vi "Get Name Filtered Categories.vi"(8 "error in (no error)":errorcluster, 10 "Name filter":string, 11 "Database in":refnum<class "Account History.lvclass">) -> (0 "error out":errorcluster, 2 "Categories":refnum<class "Category.lvclass">[](array[class]), 3 "Database out":refnum<class "Account History.lvclass">)   [LabVIEW 2018, in "Account History.lvclass"]
uses:
  Account History.lvclass
  Category/Category.lvclass
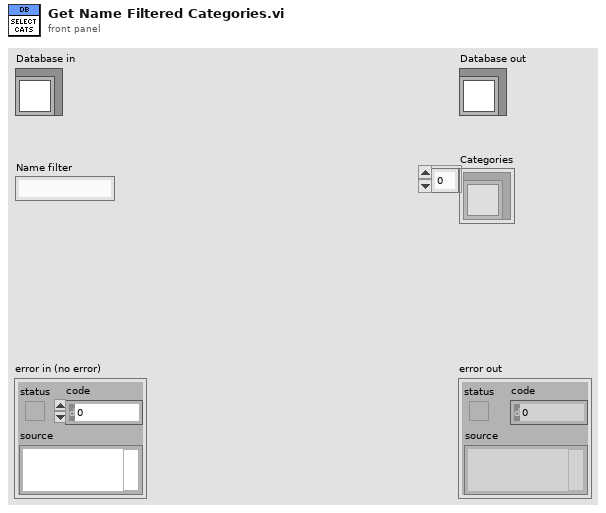
[diagram p1: front panel]
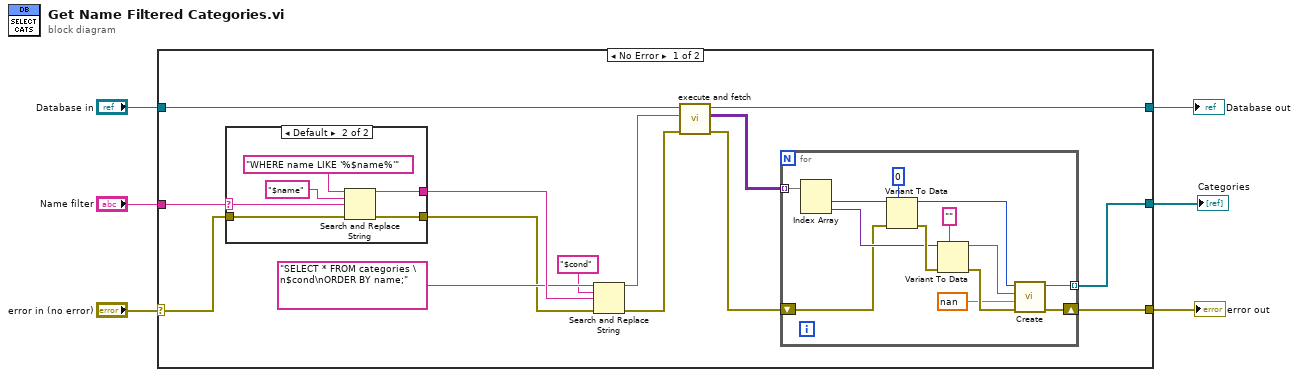
[diagram p0: block diagram]
diagram:
  n1 = case shown="No Error" "error in (no error)" {
    selector: "error in (no error)" -> [w8 w41]
    tunnel: [w13 w42] -> w6
    tunnel: "Database in" -> [w12 w42]
    tunnel: [w11 w41] -> w4
    tunnel: "Name filter" -> [w10 _]
    tunnel: [w9 _] -> w2
    frame No Error {
      n2 = case shown="Default" w10 {
        selector: w10 -> [_ w27]
        tunnel: [_ w24] -> w17
        tunnel: w8 -> [w21 w23]
        tunnel: [w21 w22] -> w7
        frame "" {
        }
        frame Default {
          n3 = Search and Replace String(input string="WHERE name LIKE '%$name%'", search string="$name", replace string=w27, error in=w23) -> (result string=w24:string, error out=w22:errorcluster)  [unwired: 4 in, 2 out]
        }
      }
      n4 = Search and Replace String(input string="SELECT * FROM categories \n$cond\nORDER BY name;", search string="$cond", replace string=w17, error in=w7) -> (result string=w14:string, error out=w18:errorcluster)  [unwired: 4 in, 2 out]
      n5 = call "execute and fetch.vi"("error in (no error)"=w18, "SQL query"=w14, "Database in"=w12) -> ("error out"=w19:errorcluster, "recordset data"=w20:variant[][], "Database out"=w13:refnum<class "Account History.lvclass">)  [unwired: 5 in, 1 out]
      n6 = for {
        tunnel: w20 -> [w33] mode=indexing
        shift-right: [w39] -> w11
        shift-left: w19 -> [w32]
        tunnel: [w40] -> w9 mode=indexing
        n7 = Index Array(array=w33) -> (element #1=w36:variant, element #2=w37:variant)  [unwired: 2 in]
        n8 = Variant To Data(error in=w32, type=0, Variant=w36) -> (data=w30:i32, error out=w38:errorcluster)
        n9 = Variant To Data(error in=w38, type="", Variant=w37) -> (data=w29:string, error out=w31:errorcluster)
        n10 = call "Create.vi"("error in (no error)"=w31, "Default Goal Amount"=nan, "Name"=w29, "id"=w30) -> ("error out"=w39:errorcluster, "Category out"=w40:refnum<class "Category.lvclass">)  [unwired: 6 in]
      }
    }
    frame Error {
    }
  }
  "error out" <- w4
  "Database out" <- w6
  "Categories" <- w2
